vi "Init.vi"(8 "error in (no error)":errorcluster, 9 "SA Pin":string, 10 "Measurement Name":string) -> (0 "error out":errorcluster, 3 "WCDMA_CHP out":refnum<class "WCDMA_CHP.lvclass">)   [LabVIEW 2016, in "SeqAuto Evaluations.lvlib" / "WCDMA_CHP.lvclass"]
uses:
  WCDMA_CHP.lvclass
  C:/Sequence Automation/Plugins/SeqAuto IEvaluation.lvlibp/SeqAuto IEvaluation.lvclass
  WCDMA_CHP.lvclass/WCDMA_CHP.ctl
  Write SA Pin.vi
  Plugins/SeqAuto IEvaluation.lvlibp/Write Measurement Name.vi
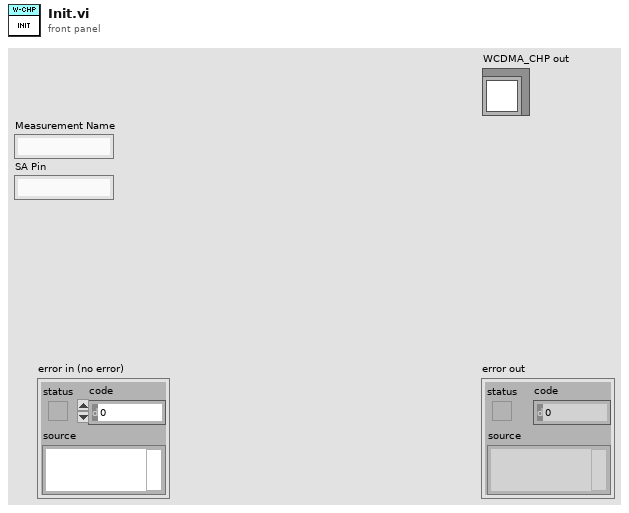
[diagram p1: front panel]
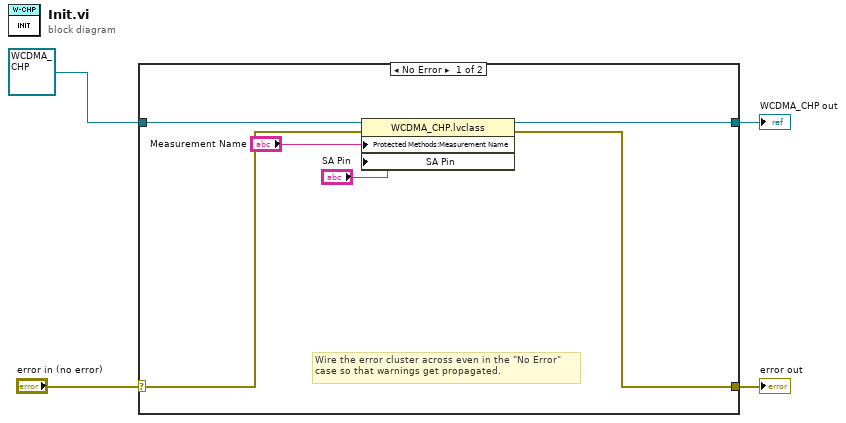
[diagram p0: block diagram]
diagram:
  n1 = case shown="No Error" "error in (no error)" {
    selector: "error in (no error)" -> [w10 w12]
    tunnel: [w9 w12] -> w3
    tunnel: [w7 w11] -> w1
    tunnel: refnum<class "WCDMA_CHP.lvclass"> refnum ("WCDMA_CHP in") -> [w8 w11]
    frame No Error {
      # "Wire the error cluster across even in the \"No Error\"\ncase so that warnings get propagated."
      n2 = property class="WCDMA_CHP.lvclass"(reference=w8, error in=w10, "Protected Methods:Measurement Name"="Measurement Name", "SA Pin"="SA Pin") -> (reference out=w7:refnum<class "WCDMA_CHP.lvclass">, error out=w9:errorcluster)
    }
    frame Error {
    }
  }
  "error out" <- w3
  "WCDMA_CHP out" <- w1
